vi "SubPanelAttach.vi"(8 "error in (no error)":errorcluster, 11 "VMUI in":refnum<class "VMUI.lvclass">) -> (0 "error out":errorcluster, 3 "VMUI out":refnum<class "VMUI.lvclass">)   [LabVIEW 2013, in "VMUI.lvclass"]
uses:
  VMUI.lvclass
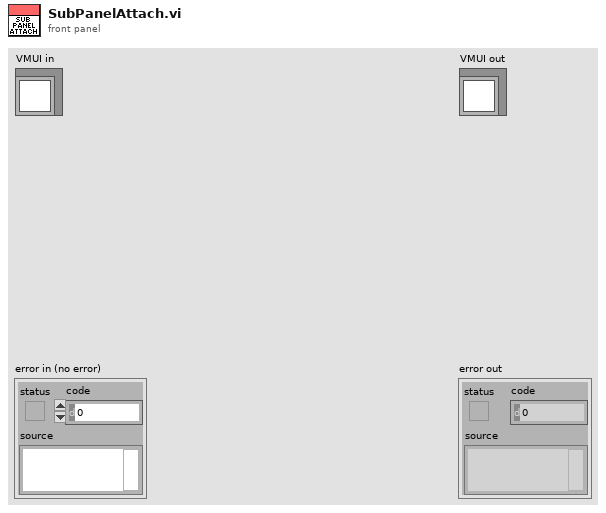
[diagram p1: front panel]
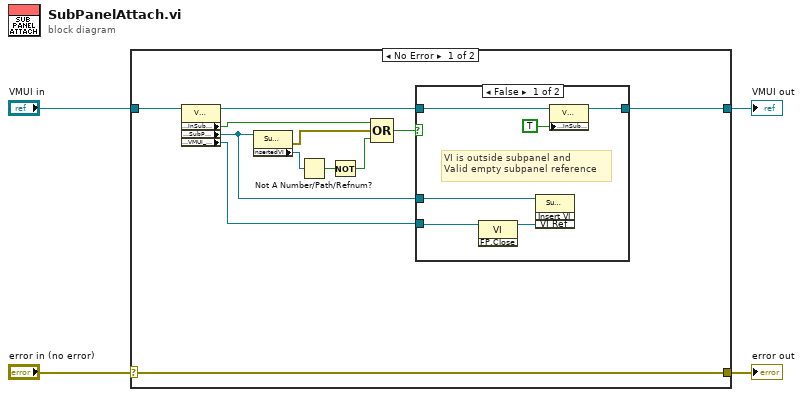
[diagram p0: block diagram]
diagram:
  n1 = case shown="No Error" "error in (no error)" {
    selector: "error in (no error)" -> [w16 w25]
    tunnel: [w16 w25] -> w3
    tunnel: [w9 w24] -> w1
    tunnel: "VMUI in" -> [w15 w24]
    frame No Error {
      n2 = property class="VMUI.lvclass"(reference=w15) -> (reference out=w10:refnum<class "VMUI.lvclass">, "Accessors:InSubPanel"=w8:bool, "Accessors:SubPanelRef"=w12:refnum<vi>, "Accessors:VMUI_VI_Ref"=w11:refnum<vi>)  [unwired: 1 in, 1 out]
      n3 = property class="SubPnl"(reference=w12) -> (error out=w7:errorcluster, "InsertedVI"=w13:refnum<vi>)  [unwired: 1 in, 1 out]
      n4 = Not A Number/Path/Refnum?(number/path/refnum=w13) -> (NaN/Path/Refnum?=w14:bool)
      n5 = Not(x=w14) -> (.not. x?=w6:bool)
      n6 = Compound Arithmetic op=OR(w8, w7, w6) -> (w5:bool)
      n7 = case shown="False" w5 {
        tunnel: w11 -> [w22 _]
        tunnel: w12 -> [w20 _]
        tunnel: w10 -> [w19 w23]
        tunnel: [w18 w23] -> w9
        frame False {
          # "VI is outside subpanel and\nValid empty subpanel reference"
          n8 = invoke class="VI" method="FP.Close"(reference=w22) -> (reference out=w21:refnum<vi>)  [unwired: 2 in, 2 out]
          n9 = invoke class="SubPnl" method="Insert VI"(reference=w20, "VI Ref"=w21) -> ()  [unwired: 2 in, 4 out]
          n10 = property class="VMUI.lvclass"(reference=w19, "Accessors:InSubPanel"=TRUE) -> (reference out=w18:refnum<class "VMUI.lvclass">)  [unwired: 1 in, 1 out]
        }
        frame True {
          # "VI is already inside a subpanel, or\nInvalid subpanel reference, or\nreferenced subpanel is occupied"
        }
      }
    }
    frame Error {
    }
  }
  "error out" <- w3
  "VMUI out" <- w1
